vi "Overlay Circle.vi"(4 "Color":u32(colorbox)=16711680, 6 "Size":sgl, 8 "error in (no error)":errorcluster, 9 "point":cluster{"X [px]":sgl, "Y [px]":sgl}, 11 "Image In":T1) -> (0 "error out":errorcluster, 3 "Image Out":T1(plugin-control))   [LabVIEW 2023, in "Camera Calibration.lvlib"]
uses:
  <vilib>/vision/Image Controls.llb/IMAQ Image.ctl
  Camera Calibration.lvlib
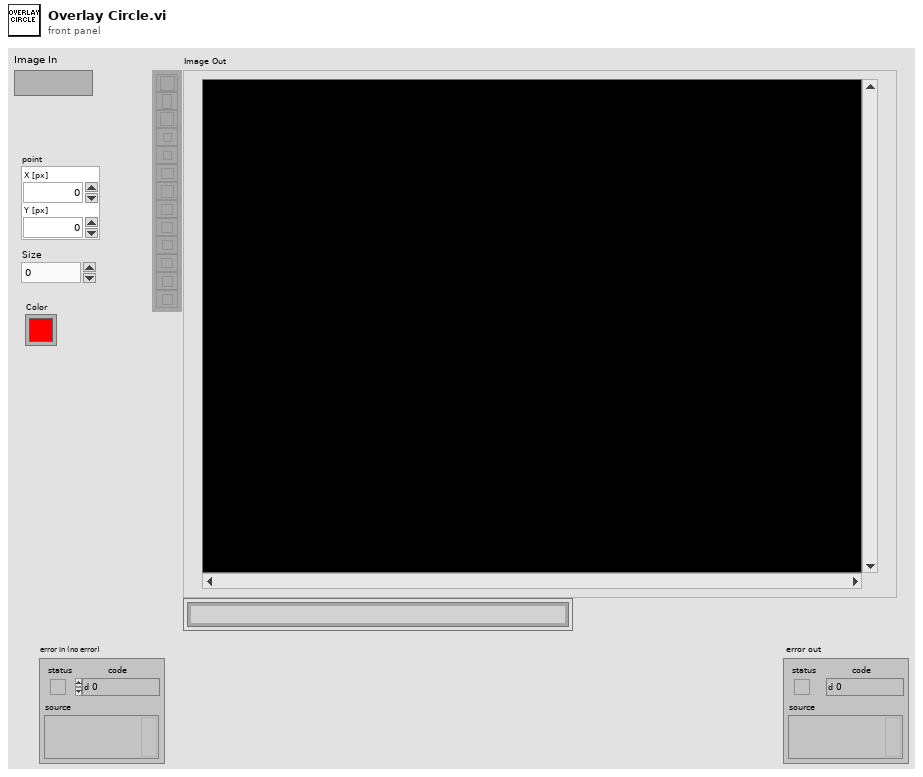
[diagram p1: front panel]
types:
  T1 = typedef "IMAQ Image.ctl" = refnum<image>
  T2 = cluster{"Left":i32, "Top":i32, "Right":i32, "Bottom":i32}
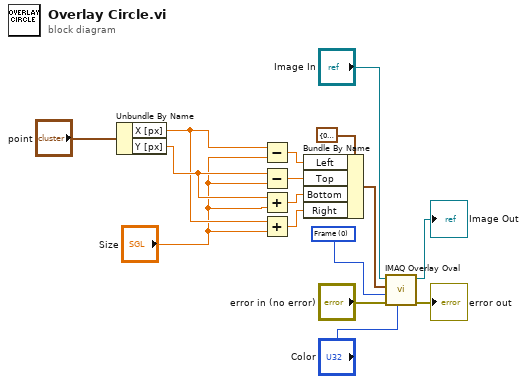
[diagram p0: block diagram]
diagram:
  w10 = u32 0 items=["Frame", "Fill"] ("Drawing Mode (Frame)")
  n1 = Unbundle By Name("point") -> ("X [px]"=w3:sgl, "Y [px]"=w4:sgl)
  n2 = Subtract(x=w3, y="Size") -> (x-y=w15:sgl)
  n3 = Subtract(x=w4, y="Size") -> (x-y=w14:sgl)
  n4 = Add(x=w4, y="Size") -> (x+y=w13:sgl)
  n5 = Add(x=w3, y="Size") -> (x+y=w12:sgl)
  n6 = Bundle By Name(cluster=T2 {"Left"=0, "Top"=0, "Right"=0, "Bottom"=0} ("Bounding Rectangle"), "Left"=w15, "Top"=w14, "Bottom"=w13, "Right"=w12) -> (w1:T2)
  n7 = call "IMAQ Overlay Oval"("Color"="Color", "error in (no error)"="error in (no error)", "Drawing Mode (Frame)"=w10, "Bounding Rectangle"=w1, "Image"="Image In") -> ("error out"=→"error out":errorcluster, "Image Out"=→"Image Out":T1)  [unwired: 5 in]
